vi "TEMOCR-Initialize SGDA.vi"(0 "Data folder":path, 5 "Params":T2, 11 "error in (no error)":errorcluster) -> (3 "Num Levels":i32, 4 "AO":T1, 15 "error out":errorcluster)   [LabVIEW 2015]
uses:
  Typedefs/TEMOCR-Parameters.ctl
  Typedefs/TEMOCR-Probe.ctl
  Typedefs/TEMOCR-Elicitor.ctl
  Human Studies/SFM Frontend/LV Source/Typedefs/HSTS-Transducer.ctl
  Typedefs/TEMOCR-Sequence.ctl
  Typedefs/TEMOCR-Analysis.ctl
  Typedefs/TEMOCR-AO Data.ctl
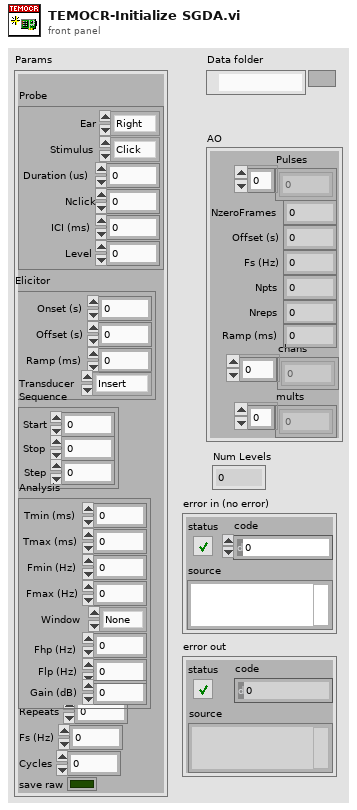
[diagram p1: front panel]
types:
  T1 = typedef "TEMOCR-AO Data.ctl" = cluster{"Pulses":dbl[], "Fs (Hz)":dbl, "Npts":i32, "mults":dbl[], "chans":i32[], "Nreps":i32, "NzeroFrames":i32, "Offset (s)":dbl, "Ramp (ms)":dbl}
  T2 = typedef "TEMOCR-Parameters.ctl" = cluster{"Probe":T3, "Elicitor":T4, "Sequence":T6, "Analysis":T7, "Repeats":i32, "Fs (Hz)":dbl, "Cycles":i32, "save raw":bool}
  T3 = typedef "TEMOCR-Probe.ctl" = cluster{"Ear":enum16{"Right", "Left"}, "Stimulus":enum16{"Click", "Chirp"}, "Duration (us)":dbl, "Nclick":i32, "ICI (ms)":dbl, "Level":dbl}
  T4 = typedef "TEMOCR-Elicitor.ctl" = cluster{"Onset (s)":dbl, "Offset (s)":dbl, "Ramp (ms)":dbl, "Transducer":T5}
  T5 = typedef "HSTS-Transducer.ctl" = enum16{"Insert", "TDH-39", "HD300", "ER-10X"}
  T6 = typedef "TEMOCR-Sequence.ctl" = cluster{"Start":dbl, "Stop":dbl, "Step":dbl}
  T7 = typedef "TEMOCR-Analysis.ctl" = cluster{"Tmin (ms)":dbl, "Tmax (ms)":dbl, "Fmin (Hz)":dbl, "Fmax (Hz)":dbl, "Window":enum16{"None", "Hanning", "Hamming"}, "Fhp (Hz)":dbl, "Flp (Hz)":dbl, "Gain (dB)":dbl}
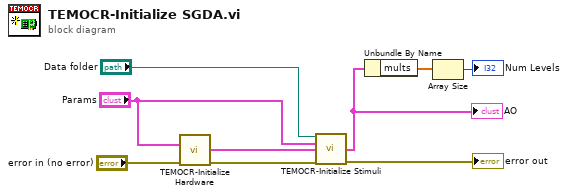
[diagram p0: block diagram]
diagram:
  n1 = call "TEMOCR-Initialize Hardware.vi"("Params"="Params", "error in (no error)"="error in (no error)") -> ("AO"=w7:T1, "error out"=w6:errorcluster)  [unwired: 12 in]
  n2 = call "TEMOCR-Initialize Stimuli.vi"("Data folder"="Data folder", "Params"="Params", "AO in"=w7, "error in (no error)"=w6) -> ("AO out"=w3:T1, "error out"=→"error out":errorcluster)  [unwired: 10 in]
  "AO" <- w3
  n3 = Unbundle By Name(w3) -> ("mults"=w2:dbl[])
  n4 = Array Size(array=w2) -> (size(s)=→"Num Levels":i32)
